vi "Get error from National Instruments error.vi"(2 "Window Title":string, 11 "error out":errorcluster, 13 "String":string) -> ()   [LabVIEW 2020]
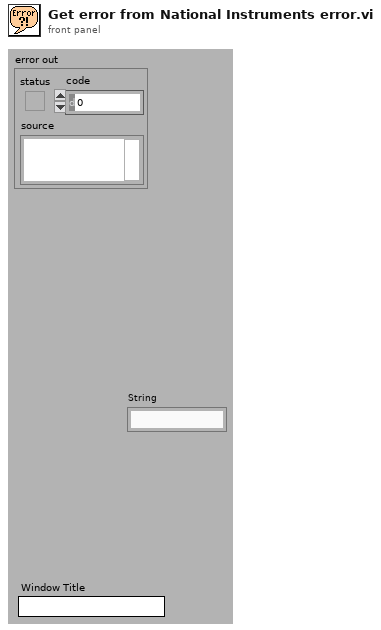
[diagram p1: front panel]
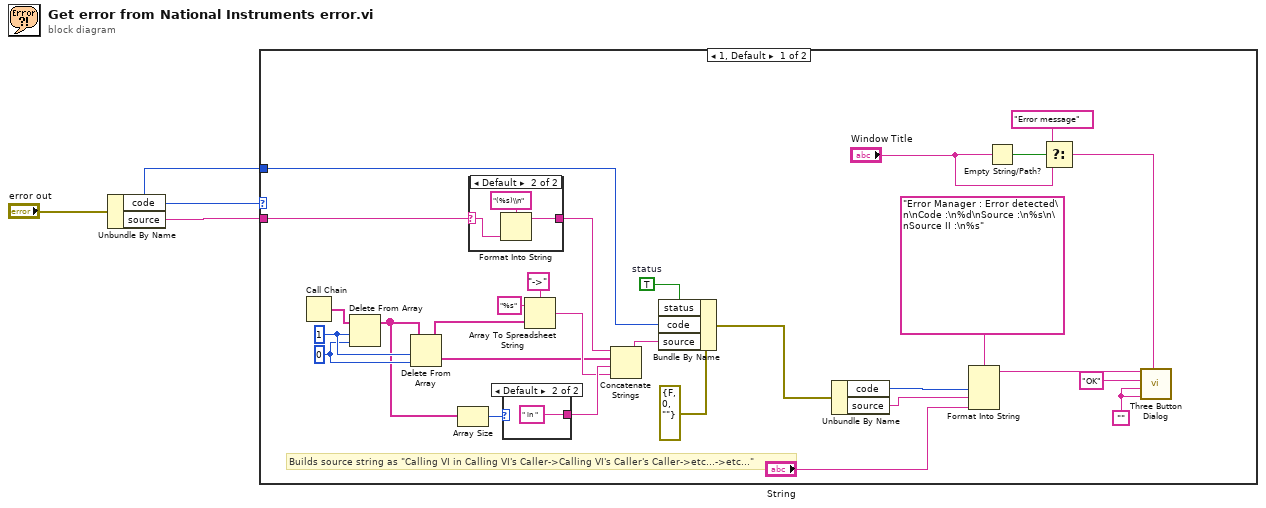
[diagram p0: block diagram]
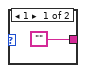
[diagram p2: hidden frame]
diagram:
  n1 = Unbundle By Name("error out") -> ("code"=w2:i32, "source"=w1:string)
  n2 = case shown="1, Default" w2 {
    tunnel: w2 -> [w19 _]
    tunnel: w1 -> [w17 _]
    frame 1, Default {
      w6 = ""
      w27 = 0 ("Index")
      w28 = 1 ("Length")
      w24 = TRUE  # status
      # "Builds source string as \"Calling VI in Calling VI's Caller->Calling VI's Caller's Caller->etc...->etc...\""
      n3 = Call Chain() -> (call chain=w18:string[])
      n4 = Delete From Array(array=w18, length=w28, index=w27) -> (array with subset deleted=w16:string[])  [unwired: 1 out]
      n5 = Delete From Array(array=w16, length=w28, index=w27) -> (deleted portion=w20:string[], array with subset deleted=w26:string[])
      n6 = Array Size(array=w16) -> (size(s)=w21:i32)
      n7 = case shown="Default" w17 {
        selector: w17 -> [w35 w38]
        tunnel: [w35 w36] -> w22
        frame "" {
        }
        frame Default {
          n8 = Format Into String(format string="(%s)\\n" ("Format String"), w38) -> (resulting string=w36:string)  [unwired: 2 in, 1 out]
        }
      }
      n9 = case shown="Default" w21 {
        tunnel: ["" " in " ("Format String")] -> w31
        frame 1 {
        }
        frame Default {
        }
      }
      n10 = Array To Spreadsheet String(delimiter (Tab)="->", array=w26, 3:"%s" ("format string")) -> (spreadsheet string=w30:string)
      n11 = Concatenate Strings(w22, w20, w31, w30) -> (w23:string)
      n12 = Bundle By Name(cluster=errorcluster {"status"=FALSE, "code"=0, "source"=""} ("error out"), "status"=w24, "code"=w19, "source"=w23) -> (w12:errorcluster)
      n13 = Unbundle By Name(w12) -> ("code"=w14:i32, "source"=w13:string)
      n14 = Format Into String(format string="Error Manager : Error detected\n\nCode :\n%d\nSource :\n%s\n\nSource II :\n%s", w14, w13, "String") -> (resulting string=w4:string)  [unwired: 2 in, 1 out]
      n15 = Empty String/Path?(string/path="Window Title") -> (empty?=w7:bool)
      n16 = Select(t="Error message", s=w7, f="Window Title") -> (s? t:f=w10:string)
      n17 = call "Three Button Dialog.vi"("Window Title (\"\")"=w10, "Right Button Text (\"Cancel\")"=w6, "Center Button Text (\"No\")"=w6, "Left Button Text (\"Yes\")"="OK" ("Left Button Text (\"Yes\")"), "message"=w4) -> ()  [unwired: 6 in, 1 out]
    }
    frame 0 {
    }
  }
